vi "counter_mod_n.vi"(9 "bool":bool, 10 "n":u8) -> (1 "sum":u8)   [LabVIEW 2018]
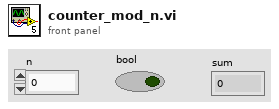
[diagram p1: front panel]
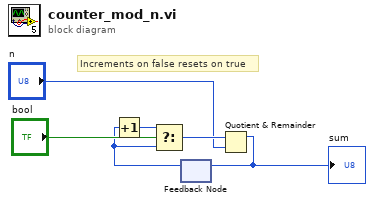
[diagram p0: block diagram]
diagram:
  # "Increments on false resets on true"
  n1 = feedback #1() -> (w2:u8)  [unwired: 1 in]
  n2 = Increment(x=w2) -> (x+1=w1:u8)
  n3 = Select(t=w1, s="bool", f=w2) -> (s? t:f=w5:u8)
  n4 = Quotient & Remainder(x=w5, y="n") -> (x-y*floor(x/y)=w3:u8)  [unwired: 1 out]
  "sum" <- w3
  n5 = feedback-in #1(w3) -> ()
